vi "Send Data to Robot.vi"(8 "error in (no error)":errorcluster, 10 "String":string, 11 "UR5 Robot in":refnum<class "UR5 Robot.lvclass">) -> (0 "error out":errorcluster, 3 "UR5 Robot out":refnum<class "UR5 Robot.lvclass">)   [LabVIEW 2018, in "UR5 Robot.lvlib" / "UR5 Robot.lvclass"]
uses:
  UR5 Robot.lvclass
  UR5 Robot.lvclass/UR5 Robot.ctl
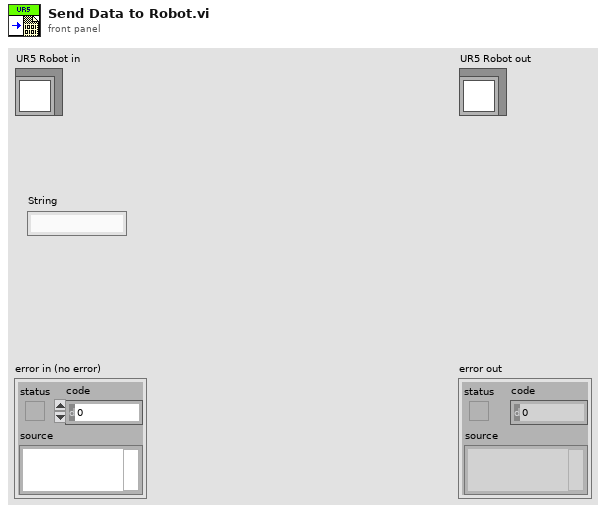
[diagram p1: front panel]
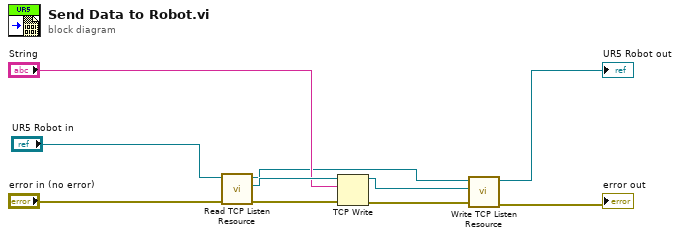
[diagram p0: block diagram]
diagram:
  n1 = call "Read TCP Listen Resource.vi"("error in (no error)"="error in (no error)", "UR5 Robot in"="UR5 Robot in") -> ("error out"=w7:errorcluster, "TCP Listen Resource"=w8:refnum<k5>, "UR5 Robot out"=w4:refnum<class "UR5 Robot.lvclass">)  [unwired: 7 in]
  n2 = TCP Write(connection ID=w8, data in="String", error in (no error)=w7) -> (connection ID out=w5:refnum<k5>, error out=w3:errorcluster)  [unwired: 1 in, 1 out]
  n3 = call "Write TCP Listen Resource.vi"("error in (no error)"=w3, "TCP Listen Resource"=w5, "UR5 Robot in"=w4) -> ("error out"=→"error out":errorcluster, "UR5 Robot out"=→"UR5 Robot out":refnum<class "UR5 Robot.lvclass">)  [unwired: 7 in]
